vi "Load Configuration From File.vi"(8 "error in (no error)":errorcluster, 9 "Name (Instance)":string, 10 "Configuration Path":path, 11 "Comp Trace Controller in":refnum<class "Comp Trace Controller.lvclass">) -> (0 "error out":errorcluster, 2 "Unflattened":string, 3 "Comp Trace Controller out":refnum<class "Comp Trace Controller.lvclass">)   [LabVIEW 2014, in "Comp Trace Controller.lvlib" / "Comp Trace Controller.lvclass"]
uses:
  Comp Trace Controller.lvclass
  Robot Actor Framework/Trace/Trace Controller Class/Trace Controller.lvclass
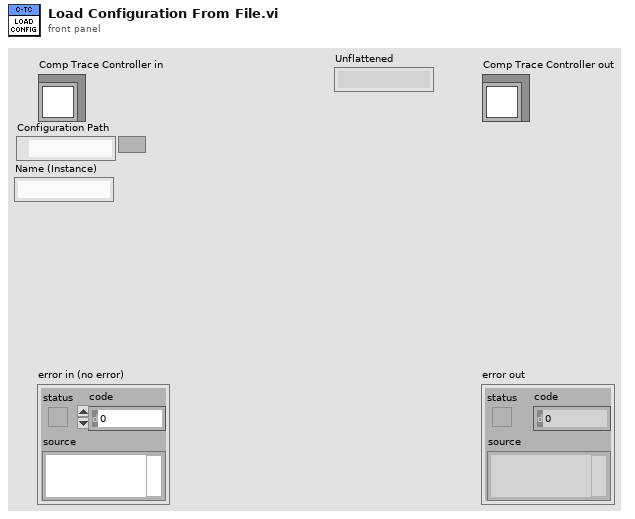
[diagram p1: front panel]
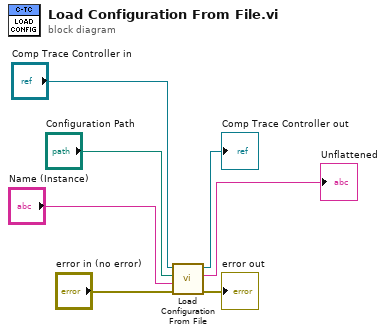
[diagram p0: block diagram]
diagram:
  n1 = call-parent "Load Configuration From File.vi"("error in (no error)"="error in (no error)", "Name (Instance)"="Name (Instance)", "Configuration Path"="Configuration Path", "System Actor in"="Comp Trace Controller in") -> ("error out"=→"error out":errorcluster, "Unflattened"=→"Unflattened":string, "System Actor out"=→"Comp Trace Controller out":refnum<class "Comp Trace Controller.lvclass">)  [unwired: 5 in]
